vi "设定参数对话框.vi"(11 "获取参数(定点数)":T1) -> (1 "参数 2":u16=3000, 2 "设定参数（定点数）选择 2":T2(ring), 3 "确定?":bool)   [LabVIEW 2016, in "环境动力监测库.lvlib" / "空调库.lvlib"]
panel:
  in  "参数":u16=3000
  in  "设定参数（定点数）选择":T2(ring)
  in  "取消":bool
  in  "确定":bool
  # "设定参数选择"
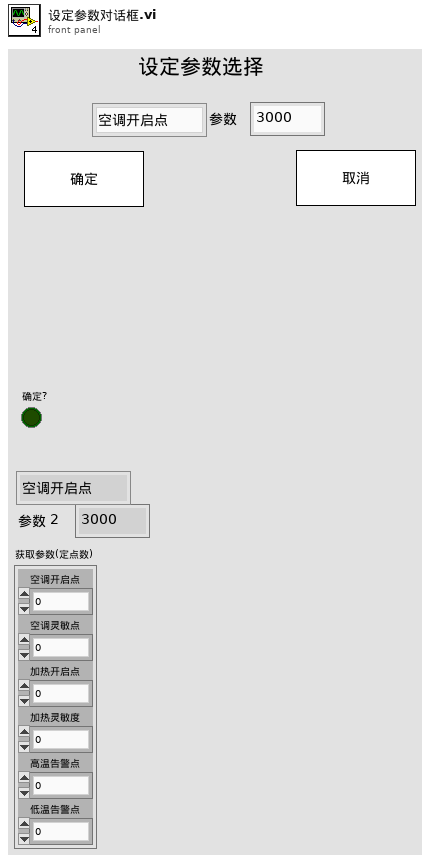
[diagram p1: front panel]
types:
  T1 = cluster{"空调开启点":u16, "空调灵敏点":u16, "加热开启点":u16, "加热灵敏度":u16, "高温告警点":u16, "低温告警点":u16}
  T2 = enum16{"空调开启点", "空调灵敏点", "加热开启点", "加热灵敏度", "高温告警点", "低温告警点"}
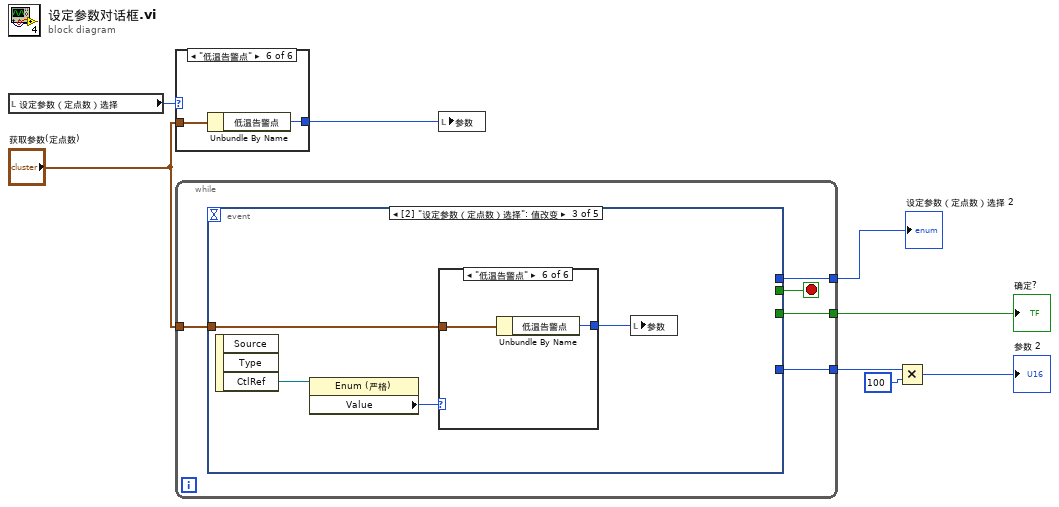
[diagram p0: block diagram]
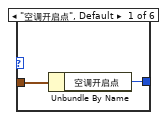
[diagram p2: hidden frame]
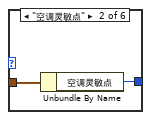
[diagram p3: hidden frame]
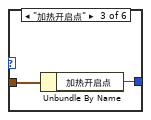
[diagram p4: hidden frame]
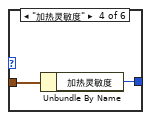
[diagram p5: hidden frame]
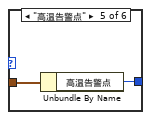
[diagram p6: hidden frame]
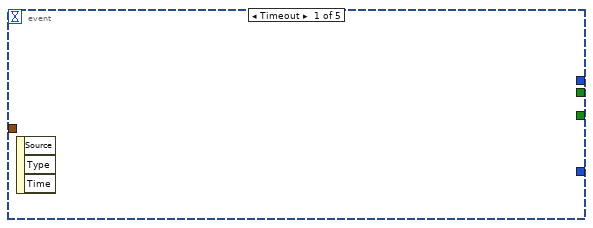
[diagram p7: hidden frame]
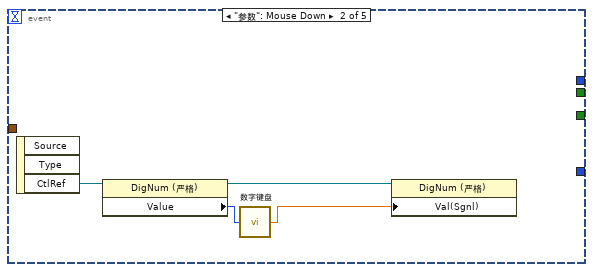
[diagram p8: hidden frame]
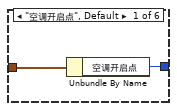
[diagram p9: hidden frame]
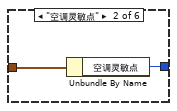
[diagram p10: hidden frame]
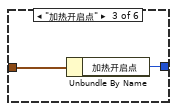
[diagram p11: hidden frame]
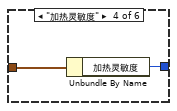
[diagram p12: hidden frame]
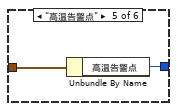
[diagram p13: hidden frame]
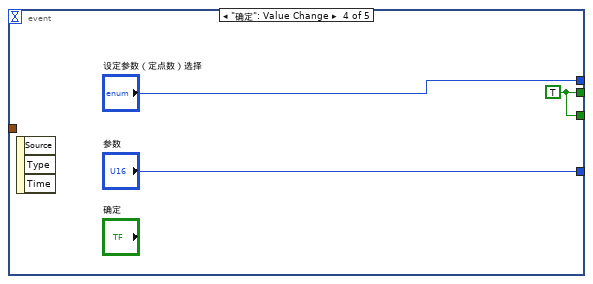
[diagram p14: hidden frame]
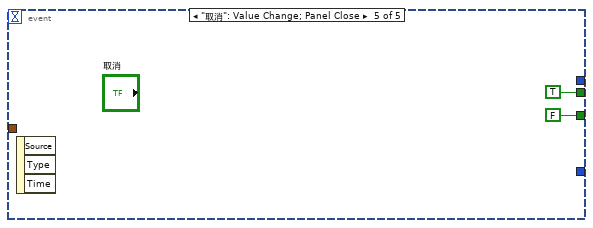
[diagram p15: hidden frame]
diagram:
  n1 = local read "设定参数（定点数）选择"() -> (w3:T2)
  n2 = case shown="\"低温告警点\"" w3 {
    tunnel: "获取参数(定点数)" -> [w10 w12 w14 w16 w18 w20]
    tunnel: [w9 w11 w13 w15 w17 w19] -> w1
    frame "空调开启点", Default {
      n3 = Unbundle By Name(w10) -> ("空调开启点"=w9:u16)
    }
    frame "空调灵敏点" {
      n4 = Unbundle By Name(w12) -> ("空调灵敏点"=w11:u16)
    }
    frame "加热开启点" {
      n5 = Unbundle By Name(w14) -> ("加热开启点"=w13:u16)
    }
    frame "加热灵敏度" {
      n6 = Unbundle By Name(w16) -> ("加热灵敏度"=w15:u16)
    }
    frame "高温告警点" {
      n7 = Unbundle By Name(w18) -> ("高温告警点"=w17:u16)
    }
    frame "低温告警点" {
      n8 = Unbundle By Name(w20) -> ("低温告警点"=w19:u16)
    }
  }
  n9 = while {
    tunnel: [w25] -> w6
    tunnel: [w23] -> w8
    tunnel: [w22] -> w7
    tunnel: "获取参数(定点数)" -> [w21]
    stop <- w24 stop-if-true
    n10 = event shown="[2] \"设定参数（定点数）选择\": 值改变" {
      selector: _ -> [_ _ _ _ _]
      dyn-events: _ -> [_ _ _ _ _]
      timeout: _ -> [_ _ _ _ _]
      tunnel: [_ _ _ w48 TRUE] -> w24
      tunnel: [_ _ _ "参数" _] -> w25
      tunnel: [_ _ _ w48 FALSE] -> w23
      tunnel: [_ _ _ "设定参数（定点数）选择" _] -> w22
      tunnel: w21 -> [_ _ w31 _ _]
      event Timeout {
        n11 = event-data() -> ()  [unwired: 1 in, 3 out]
      }
      event "参数": Mouse Down {
        n12 = event-data() -> ("CtlRef"=w29:refnum<vi>)  [unwired: 1 in, 2 out]
        n13 = property class="DigNum (严格)"(reference=w29) -> (reference out=w26:refnum<vi>, "Value"=w28:u16)  [unwired: 1 in, 1 out]
        n14 = call "数字键盘.vi"("OldNumber"=w28) -> ("NewNumber"=w27:sgl)
        n15 = property class="DigNum (严格)"(reference=w26, "Val(Sgnl)"=w27) -> ()  [unwired: 1 in, 2 out]
      }
      event "设定参数（定点数）选择": Value Change {
        n16 = event-data() -> ("CtlRef"=w33:refnum<vi>)  [unwired: 1 in, 2 out]
        n17 = property class="Enum (严格)"(reference=w33) -> ("Value"=w32:T2)  [unwired: 1 in, 2 out]
        n18 = case shown="\"低温告警点\"" w32 {
          tunnel: w31 -> [w35 w37 w39 w41 w43 w45]
          tunnel: [w34 w36 w38 w40 w42 w44] -> w30
          frame "空调开启点", Default {
            n19 = Unbundle By Name(w35) -> ("空调开启点"=w34:u16)
          }
          frame "空调灵敏点" {
            n20 = Unbundle By Name(w37) -> ("空调灵敏点"=w36:u16)
          }
          frame "加热开启点" {
            n21 = Unbundle By Name(w39) -> ("加热开启点"=w38:u16)
          }
          frame "加热灵敏度" {
            n22 = Unbundle By Name(w41) -> ("加热灵敏度"=w40:u16)
          }
          frame "高温告警点" {
            n23 = Unbundle By Name(w43) -> ("高温告警点"=w42:u16)
          }
          frame "低温告警点" {
            n24 = Unbundle By Name(w45) -> ("低温告警点"=w44:u16)
          }
        }
        n25 = local write "参数"(w30) -> ()
      }
      event "确定": Value Change {
        w48 = TRUE
        n26 = event-data() -> ()  [unwired: 1 in, 3 out]
      }
      event "取消": Value Change; Panel Close {
        n27 = event-data() -> ()  [unwired: 1 in, 3 out]
      }
    }
  }
  "确定?" <- w8
  "设定参数（定点数）选择 2" <- w7
  n28 = local write "参数"(w1) -> ()
  n29 = Multiply(x=w6, y=u16 100) -> (x*y=→"参数 2":u16)
